vi "Event Create Once.vi"(7 "ini":bool) -> (3 "Camera Events":refnum<user-event>, 4 "Camera Events 2":T1={"Event Type"=enum."Save Data", "Setpoint"=100, "Camera"="", "Video Modes"=[]})   [LabVIEW 2023]
uses:
  Ctrl/Camera Event Cluster.ctl
  Event Setup Types.ctl
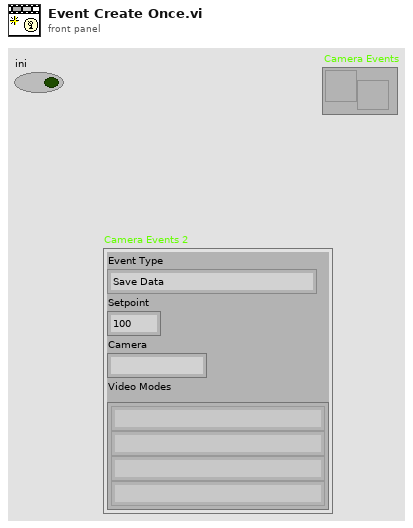
[diagram p1: front panel]
types:
  T1 = typedef "Camera Event Cluster.ctl" = cluster{"Event Type":T2, "Setpoint":i64, "Camera":string, "Video Modes":string[]}
  T2 = typedef "Event Setup Types.ctl" = enum16{"Default", "Camera Loop Started", "Close Settings", "GreyScale", "Open Front Panel", "Reset Team Number", "Save Data", "Exit"}
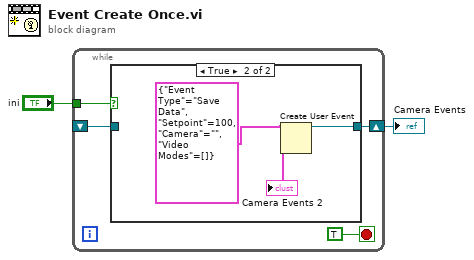
[diagram p0: block diagram]
diagram:
  n1 = while {
    shift-right: [w5] -> w2
    shift-left: _ -> [w4]
    tunnel: "ini" -> [w3]
    stop <- TRUE stop-if-true
    n2 = case shown="True" w3 {
      tunnel: [w7 w9] -> w5
      tunnel: w4 -> [w7 _]
      frame False {
      }
      frame True {
        w8 = T1 {"Event Type"=enum."Save Data", "Setpoint"=100, "Camera"="", "Video Modes"=[]} ("Camera Events")
        n3 = Create User Event(user event datatype=w8) -> (user event=w9:refnum<user-event>)  [unwired: 1 in, 1 out]
        "Camera Events 2" <- w8
      }
    }
  }
  "Camera Events" <- w2
